vi "ep_Curve Error Check.vi"(8 "error in (no error)":errorcluster, 10 "GD":u16=25, 11 "time dial":dbl=1.0) -> (0 "error out":errorcluster)   [LabVIEW 2012, in "NI_EP_Protection.lvlib"]
uses:
  <vilib>/addons/Electrical Power/Protection/NI_EP_Protection.lvlib
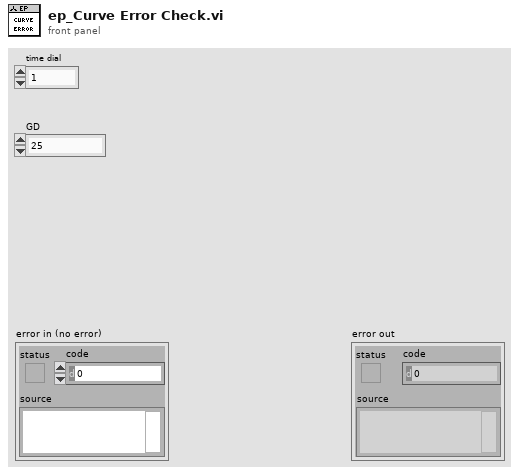
[diagram p1: front panel]
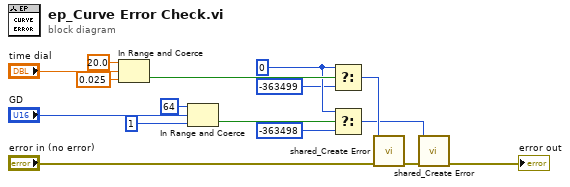
[diagram p0: block diagram]
diagram:
  w9 = 0 ("error code (0)")
  n1 = In Range and Coerce(upper limit=20.0, x="time dial", lower limit=0.025) -> (In Range?=w13:bool)  [unwired: 1 out]
  n2 = In Range and Coerce(upper limit=u16 64, x="GD", lower limit=u16 1 ("y")) -> (In Range?=w6:bool)  [unwired: 1 out]
  n3 = Select(t=w9, s=w13, f=-363499 ("error code (0)")) -> (s? t:f=w12:i32)
  n4 = Select(t=w9, s=w6, f=-363498 ("error code (0)")) -> (s? t:f=w10:i32)
  n5 = call <vilib>:"shared_Create Error.vi"("error in (no error)"="error in (no error)", "error code (0)"=w12) -> ("error out"=w11:errorcluster)  [unwired: 9 in]
  n6 = call <vilib>:"shared_Create Error.vi"("error in (no error)"=w11, "error code (0)"=w10) -> ("error out"=→"error out":errorcluster)  [unwired: 9 in]
